vi "6221_2182A_one time_PD_read with small delta current.vi"(1 "6221":refnum<visa-resource-name>, 2 "Amplitude (A)":dbl=0.05, 3 "Duration (s)":dbl=5e-05, 4 "Pulse number":dbl=1.0, 5 "错误输入（无错误）":errorcluster, 7 "Reading current (A)":dbl=0.05) -> (15 "电流源地址输出":refnum<visa-resource-name>, 16 "R (mOhm)":dbl, 17 "错误输出（无错误）":errorcluster, 19 "电压（mV）":dbl[](array[numeric]))   [LabVIEW 2021]
uses:
  <vilib>/Analysis/baseanly.llb/Mean (DBL).vi
  <vilib>/Analysis/NI_AALBase.lvlib
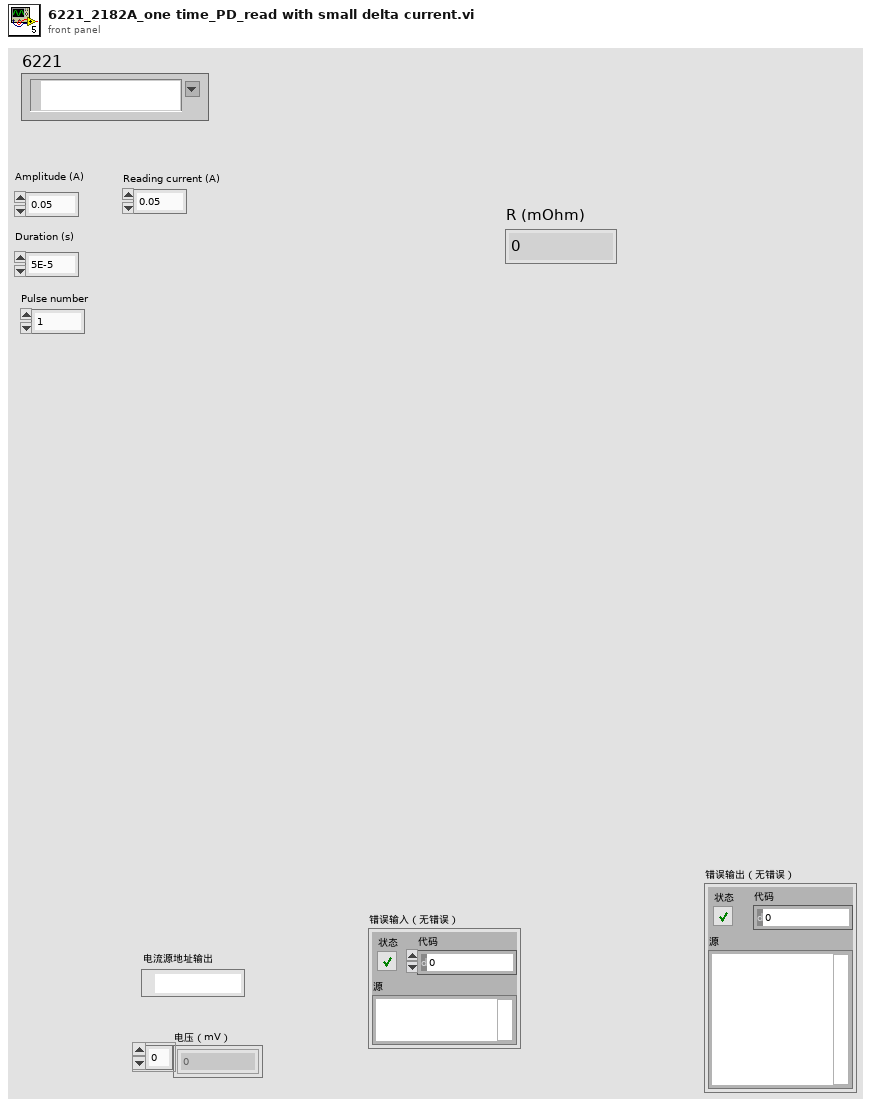
[diagram p1: front panel]
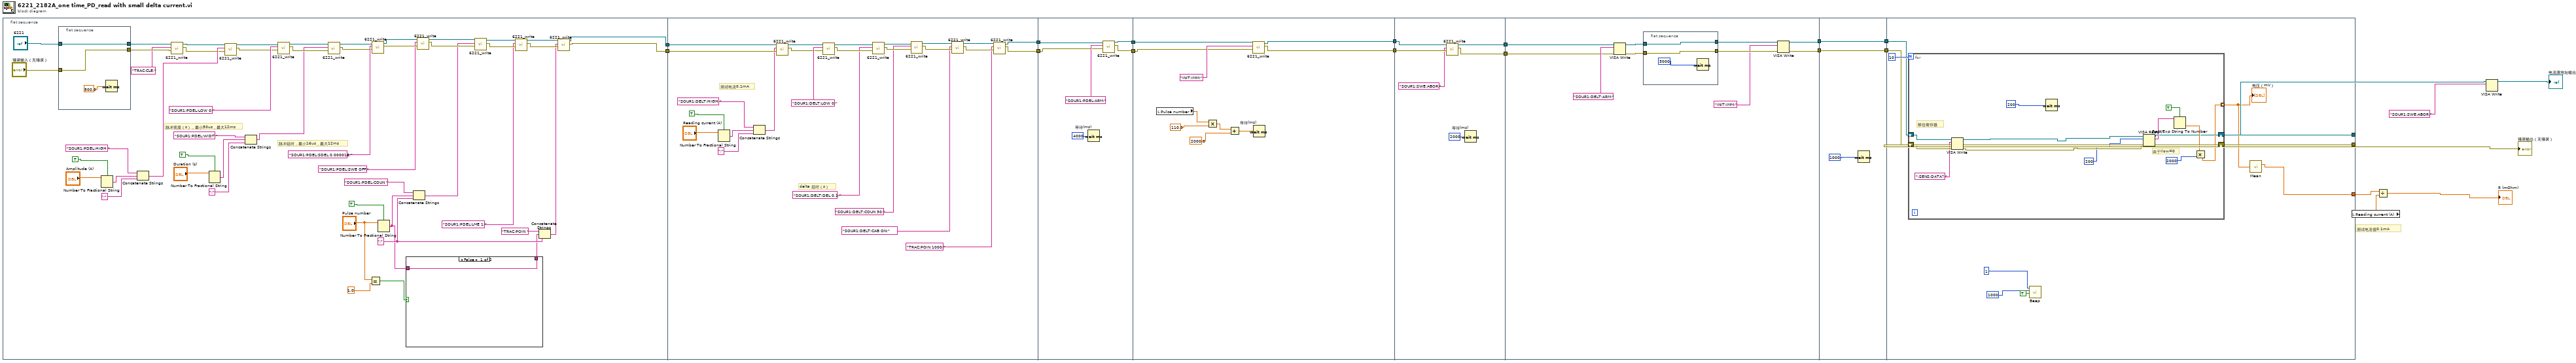
[diagram p0: block diagram]
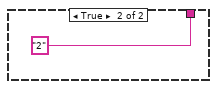
[diagram p2: hidden frame]
diagram:
  # "测试电流值0.1mA"
  n1 = flat-sequence {
    tunnel: [w38] -> w3
    tunnel: [w37] -> w2
    tunnel: [w86] -> w5
    tunnel: [w85] -> w4
    tunnel: w3 -> [w84]
    tunnel: w2 -> [w83]
    tunnel: [w104] -> w7
    tunnel: [w103] -> w6
    tunnel: w5 -> [w106]
    tunnel: w4 -> [w105]
    tunnel: [w113] -> w20
    tunnel: [w114] -> w19
    tunnel: w7 -> [w117]
    tunnel: w6 -> [w115]
    tunnel: w20 -> [w122]
    tunnel: w19 -> [w123]
    tunnel: [w120] -> w14
    tunnel: [w119] -> w13
    tunnel: [w128] -> w18
    tunnel: [w129] -> w16
    tunnel: w14 -> [w125]
    tunnel: w13 -> [w124]
    tunnel: w18 -> [w139]
    tunnel: [w139] -> w17
    tunnel: w16 -> [w138]
    tunnel: [w138] -> w15
    tunnel: w17 -> [w146]
    tunnel: w15 -> [w143]
    tunnel: [w148] -> w10
    tunnel: [w147] -> w21
    tunnel: [w145] -> w12
    frame #0 {
      w33 = ";"
      # "脉冲延时，最小16us，最大12ms"
      # "脉冲宽度（s），最小50us，最大12ms"
      n2 = flat-sequence {
        tunnel: [w76] -> w29
        tunnel: "6221" -> [w76]
        tunnel: [w75] -> w28
        tunnel: "错误输入（无错误）" -> [w75]
        frame #0 {
          n3 = Wait (ms)(milliseconds to wait=500.0) -> ()  [unwired: 1 out]
        }
      }
      n4 = Number To Fractional String(use system decimal point (T)=TRUE, number="Amplitude (A)") -> (F-format string=w68:string)  [unwired: 2 in]
      n5 = Concatenate Strings("SOUR1:PDEL:HIGH ", w68, ";") -> (w61:string)
      n6 = call "6221_write.vi"("错误输入（无错误）"=w28, "写入缓冲区"="TRAC:CLE;", "VISA资源名称"=w29) -> ("错误输出"=w30:errorcluster, "VISA资源名称输出"=w31:refnum<visa-resource-name>)  [unwired: 7 in]
      n7 = Number To Fractional String(use system decimal point (T)=TRUE, number="Duration (s)") -> (F-format string=w46:string)  [unwired: 2 in]
      n8 = call "6221_write.vi"("错误输入（无错误）"=w30, "写入缓冲区"=w61, "VISA资源名称"=w31) -> ("错误输出"=w59:errorcluster, "VISA资源名称输出"=w60:refnum<visa-resource-name>)  [unwired: 7 in]
      n9 = Concatenate Strings("SOUR1:PDEL:WIDT ", w46, ";") -> (w42:string)
      n10 = call "6221_write.vi"("错误输入（无错误）"=w59, "写入缓冲区"="SOUR1:PDEL:LOW 0;", "VISA资源名称"=w60) -> ("错误输出"=w57:errorcluster, "VISA资源名称输出"=w58:refnum<visa-resource-name>)  [unwired: 7 in]
      n11 = call "6221_write.vi"("错误输入（无错误）"=w57, "写入缓冲区"=w42, "VISA资源名称"=w58) -> ("错误输出"=w54:errorcluster, "VISA资源名称输出"=w55:refnum<visa-resource-name>)  [unwired: 7 in]
      n12 = Equal?(x="Pulse number", y=1.0) -> (x = y?=w24:bool)
      n13 = call "6221_write.vi"("错误输入（无错误）"=w54, "写入缓冲区"="SOUR1:PDEL:SDEL 0.000016;", "VISA资源名称"=w55) -> ("错误输出"=w51:errorcluster, "VISA资源名称输出"=w52:refnum<visa-resource-name>)  [unwired: 7 in]
      n14 = Number To Fractional String(use system decimal point (T)=TRUE, number="Pulse number") -> (F-format string=w22:string)  [unwired: 2 in]
      n15 = case shown="False" w24 {
        tunnel: [w72 "2"] -> w23
        tunnel: w22 -> [w72 _]
        frame False {
        }
        frame True {
        }
      }
      n16 = Concatenate Strings("SOUR1:PDEL:COUN ", w22, w33) -> (w39:string)
      n17 = call "6221_write.vi"("错误输入（无错误）"=w51, "写入缓冲区"="SOUR1:PDEL:SWE OFF;", "VISA资源名称"=w52) -> ("错误输出"=w49:errorcluster, "VISA资源名称输出"=w50:refnum<visa-resource-name>)  [unwired: 7 in]
      n18 = call "6221_write.vi"("错误输入（无错误）"=w49, "写入缓冲区"=w39, "VISA资源名称"=w50) -> ("错误输出"=w64:errorcluster, "VISA资源名称输出"=w71:refnum<visa-resource-name>)  [unwired: 7 in]
      n19 = call "6221_write.vi"("错误输入（无错误）"=w64, "写入缓冲区"="SOUR1:PDEL:LME 1;", "VISA资源名称"=w71) -> ("错误输出"=w63:errorcluster, "VISA资源名称输出"=w70:refnum<visa-resource-name>)  [unwired: 7 in]
      n20 = Concatenate Strings("TRAC:POIN ", w23, w33) -> (w32:string)
      n21 = call "6221_write.vi"("错误输入（无错误）"=w63, "写入缓冲区"=w32, "VISA资源名称"=w70) -> ("错误输出"=w37:errorcluster, "VISA资源名称输出"=w38:refnum<visa-resource-name>)  [unwired: 7 in]
    }
    frame #1 {
      # "测试电流0.1mA"
      # "delta 延时（s）"
      n22 = Number To Fractional String(use system decimal point (T)=TRUE, number="Reading current (A)") -> (F-format string=w81:string)  [unwired: 2 in]
      n23 = Concatenate Strings("SOUR1:DELT:HIGH ", w81, ";") -> (w77:string)
      n24 = call "6221_write.vi"("错误输入（无错误）"=w83, "写入缓冲区"=w77, "VISA资源名称"=w84) -> ("错误输出"=w99:errorcluster, "VISA资源名称输出"=w97:refnum<visa-resource-name>)  [unwired: 7 in]
      n25 = call "6221_write.vi"("错误输入（无错误）"=w99, "写入缓冲区"="SOUR1:DELT:LOW 0;", "VISA资源名称"=w97) -> ("错误输出"=w100:errorcluster, "VISA资源名称输出"=w98:refnum<visa-resource-name>)  [unwired: 7 in]
      n26 = call "6221_write.vi"("错误输入（无错误）"=w100, "写入缓冲区"="SOUR1:DELT:DEL 0.1;", "VISA资源名称"=w98) -> ("错误输出"=w94:errorcluster, "VISA资源名称输出"=w88:refnum<visa-resource-name>)  [unwired: 7 in]
      n27 = call "6221_write.vi"("错误输入（无错误）"=w94, "写入缓冲区"="SOUR1:DELT:COUN 30;", "VISA资源名称"=w88) -> ("错误输出"=w95:errorcluster, "VISA资源名称输出"=w90:refnum<visa-resource-name>)  [unwired: 7 in]
      n28 = call "6221_write.vi"("错误输入（无错误）"=w95, "写入缓冲区"="SOUR1:DELT:CAB ON;", "VISA资源名称"=w90) -> ("错误输出"=w96:errorcluster, "VISA资源名称输出"=w92:refnum<visa-resource-name>)  [unwired: 7 in]
      n29 = call "6221_write.vi"("错误输入（无错误）"=w96, "写入缓冲区"="TRAC:POIN 1000;", "VISA资源名称"=w92) -> ("错误输出"=w85:errorcluster, "VISA资源名称输出"=w86:refnum<visa-resource-name>)  [unwired: 7 in]
    }
    frame #2 {
      n30 = Wait (ms) "等待(ms)"(milliseconds to wait=u32 4000) -> ()  [unwired: 1 out]
      n31 = call "6221_write.vi"("错误输入（无错误）"=w105, "写入缓冲区"="SOUR1:PDEL:ARM;", "VISA资源名称"=w106) -> ("错误输出"=w103:errorcluster, "VISA资源名称输出"=w104:refnum<visa-resource-name>)  [unwired: 7 in]
    }
    frame #3 {
      n32 = local read "Pulse number"() -> (w112:dbl)
      n33 = Multiply(x=w112, y=110.0) -> (x*y=w110:dbl)
      n34 = Add(x=w110, y=2000.0) -> (x+y=w109:dbl)
      n35 = call "6221_write.vi"("错误输入（无错误）"=w115, "写入缓冲区"="INIT:IMM;", "VISA资源名称"=w117) -> ("错误输出"=w113:errorcluster, "VISA资源名称输出"=w114:refnum<visa-resource-name>)  [unwired: 7 in]
      n36 = Wait (ms) "等待(ms)"(milliseconds to wait=w109) -> ()  [unwired: 1 out]
    }
    frame #4 {
      n37 = call "6221_write.vi"("错误输入（无错误）"=w122, "写入缓冲区"="SOUR1:SWE:ABOR;", "VISA资源名称"=w123) -> ("错误输出"=w119:errorcluster, "VISA资源名称输出"=w120:refnum<visa-resource-name>)  [unwired: 7 in]
      n38 = Wait (ms) "等待(ms)"(milliseconds to wait=u32 2000) -> ()  [unwired: 1 out]
    }
    frame #5 {
      n39 = VISA Write(VISA resource name=w125, write buffer="SOUR1:DELT:ARM;", error in (no error)=w124) -> (VISA resource name out=w132:refnum<visa-resource-name>, error out=w130:errorcluster)  [unwired: 1 out]
      n40 = flat-sequence {
        tunnel: [w135] -> w133
        tunnel: w132 -> [w135]
        tunnel: [w134] -> w131
        tunnel: w130 -> [w134]
        frame #0 {
          n41 = Wait (ms)(milliseconds to wait=3000) -> ()  [unwired: 1 out]
        }
      }
      n42 = VISA Write(VISA resource name=w133, write buffer="INIT:IMM;", error in (no error)=w131) -> (VISA resource name out=w129:refnum<visa-resource-name>, error out=w128:errorcluster)  [unwired: 1 out]
    }
    frame #6 {
      n43 = Wait (ms)(milliseconds to wait=1000) -> ()  [unwired: 1 out]
    }
    frame #7 {
      n44 = for {
        N: 10 -> [_]
        shift-right: [w158] -> w148
        shift-left: w143 -> [w157]
        shift-right: [w160] -> w147
        shift-left: w146 -> [w156]
        tunnel: [w151] -> w144 mode=indexing
        # "由于Ilow=0"
        # "移位寄存器"
        n45 = VISA Write(VISA resource name=w157, write buffer=":SENS:DATA?;", error in (no error)=w156) -> (VISA resource name out=w161:refnum<visa-resource-name>, error out=w154:errorcluster)  [unwired: 1 out]
        n46 = Wait (ms)(milliseconds to wait=200) -> ()  [unwired: 1 out]
        n47 = VISA Read(VISA resource name=w161, byte count=200, error in (no error)=w154) -> (VISA resource name out=w158:refnum<visa-resource-name>, read buffer=w159:string, error out=w160:errorcluster)  [unwired: 1 out]
        n48 = Fract/Exp String To Number(use system decimal point (T)=TRUE ("使用系统小数点(T)"), string=w159) -> (number=w162:dbl)  [unwired: 2 in, 1 out]
        n49 = Multiply(x=w162, y=2000) -> (x*y=w151:dbl)
      }
      "电压（mV）" <- w144
      n50 = call <vilib>:"Beep.vi"("use system alert? (T)"=TRUE, "duration (msec)"=1000, "frequency (Hz)"=1) -> ()  [unwired: 9 in]
      n51 = call-poly <vilib>:"Mean.vi"("X"=w144) -> ("mean"=w145:dbl)  [unwired: 1 out]
    }
  }
  n52 = local read "Reading current (A)"() -> (w1:dbl)
  n53 = Divide(x=w12, y=w1) -> (x/y=→"R (mOhm)":dbl)
  n54 = VISA Write(VISA resource name=w10, write buffer="SOUR1:SWE:ABOR;") -> (VISA resource name out=→"电流源地址输出":refnum<visa-resource-name>)  [unwired: 1 in, 2 out]
  "错误输出（无错误）" <- w21
